vi "Problem1.14.vi"() -> ()   [LabVIEW 2019]
panel:
  in  "Begin Button":bool
  out "Current Element mod p":dbl
  out "Current Element":dbl
  out "Prime Array":dbl[](array[numeric])
  out "p":dbl
  out "Complete":bool
  out "Initial Array":dbl[](array[numeric])
  in  "Max Number":dbl
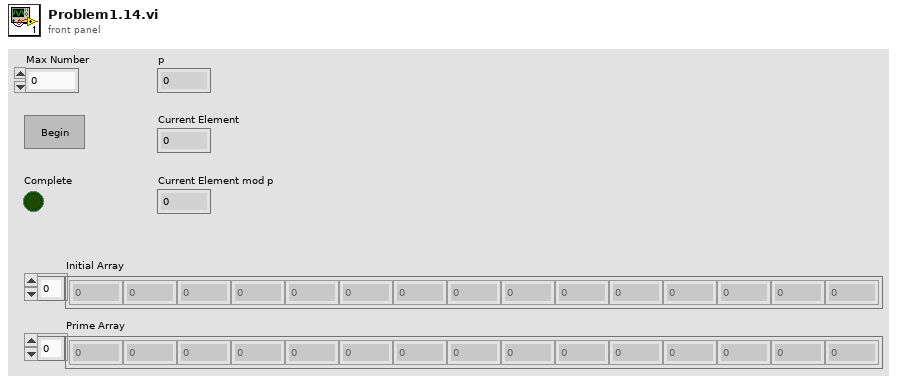
[diagram p1: front panel]
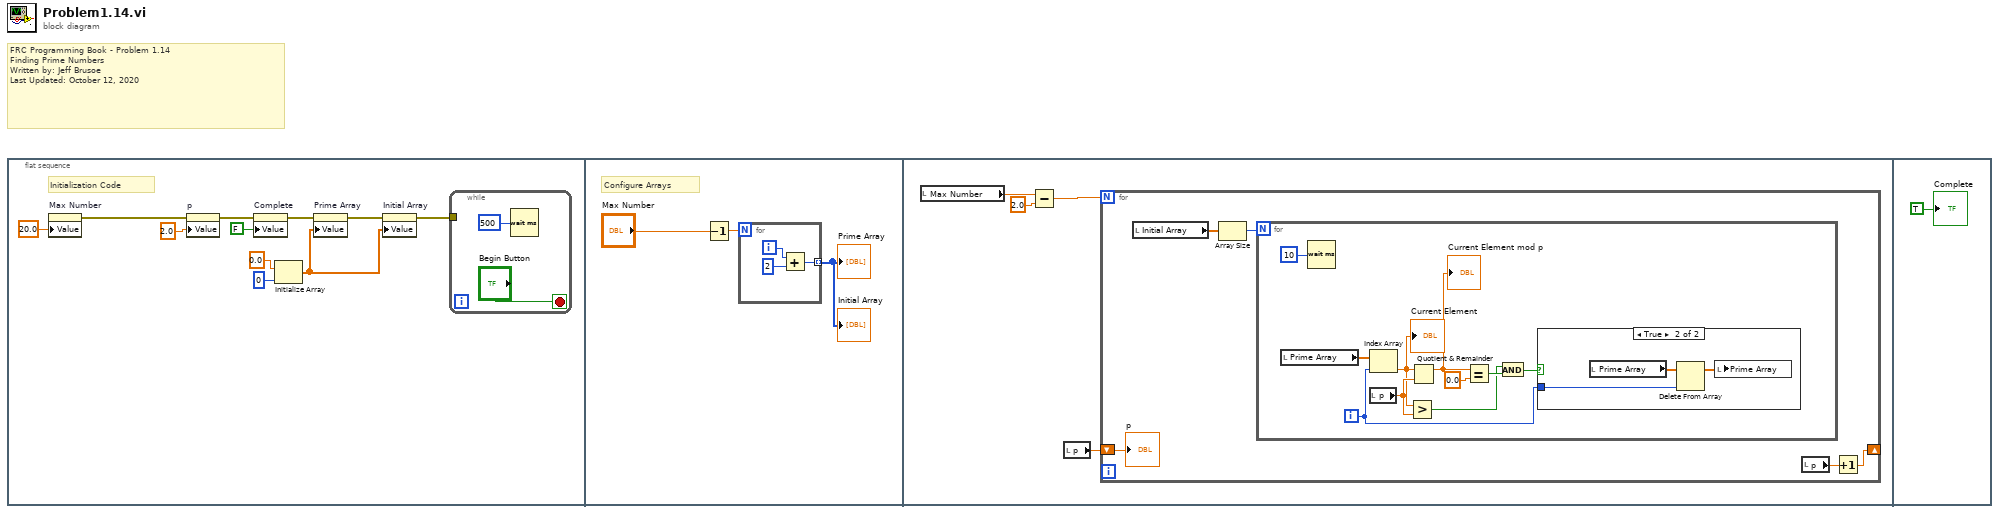
[diagram p0: block diagram]
diagram:
  # "FRC Programming Book - Problem 1.14\nFinding Prime Numbers\nWritten by: Jeff Brusoe\nLast Updated: October 12, 2020"
  n1 = flat-sequence {
    frame #0 {
      # "Initialization Code"
      n2 = property on="Max Number" class="DigNum (strict)"("Value"=20.0 ("Max Number")) -> (error out=w9:errorcluster)  [unwired: 2 in, 1 out]
      n3 = property on="p" class="DigNum (strict)"(error in=w9, "Value"=2.0 ("p")) -> (error out=w7:errorcluster)  [unwired: 1 in, 1 out]
      n4 = property on="Complete" class="Bool (strict)"(error in=w7, "Value"=FALSE ("Complete")) -> (error out=w4:errorcluster)  [unwired: 1 in, 1 out]
      n5 = Initialize Array(0.0 ("element"), 0 ("dimension size")) -> (w3:dbl[])
      n6 = property on="Prime Array" class="Arr (strict)"(error in=w4, "Value"=w3) -> (error out=w2:errorcluster)  [unwired: 1 in, 1 out]
      n7 = property on="Initial Array" class="Arr (strict)"(error in=w2, "Value"=w3) -> (error out=w1:errorcluster)  [unwired: 1 in, 1 out]
      n8 = while {
        tunnel: w1 -> [_]
        stop <- "Begin Button" stop-if-true
        n9 = Wait (ms)(milliseconds to wait=u32 500) -> ()  [unwired: 1 out]
      }
    }
    frame #1 {
      # "Configure Arrays"
      n10 = Decrement(x="Max Number") -> (x-1=w16:dbl)
      n11 = for {
        N: w16 -> [_]
        tunnel: [w17] -> w14 mode=indexing
        i -> [w19]
        n12 = Add(x=w19, y=2) -> (x+y=w17:i32)
      }
      "Initial Array" <- w14
      "Prime Array" <- w14
    }
    frame #2 {
      n13 = local read "Max Number"() -> (w21:dbl)
      n14 = Subtract(x=w21, y=2.0) -> (x-y=w22:dbl)
      n15 = local read "p"() -> (w23:dbl)
      n16 = for {
        N: w22 -> [_]
        shift-right: [w25] -> _
        shift-left: w23 -> [w26]
        n17 = local read "Initial Array"() -> (w27:dbl[])
        n18 = Array Size(array=w27) -> (size(s)=w28:i32)
        n19 = for {
          N: w28 -> [_]
          i -> [w29]
          n20 = local read "Prime Array"() -> (w38:dbl[])
          n21 = Wait (ms)(milliseconds to wait=u32 10) -> ()  [unwired: 1 out]
          n22 = Index Array(array=w38, index=w29) -> (element=w35:dbl)
          "Current Element" <- w35
          n23 = local read "p"() -> (w36:dbl)
          n24 = Greater?(x=w35, y=w36) -> (0:w31:bool)
          n25 = Quotient & Remainder(x=w35, y=w36) -> (x-y*floor(x/y)=w34:dbl)  [unwired: 1 out]
          "Current Element mod p" <- w34
          n26 = Equal?(x=w34, y=0.0) -> (x = y?=w32:bool)
          n27 = And(x=w31, y=w32) -> (x .and. y?=w30:bool)
          n28 = case shown="True" w30 {
            tunnel: w29 -> [_ w41]
            frame False {
            }
            frame True {
              n29 = local read "Prime Array"() -> (w40:dbl[])
              n30 = Delete From Array(array=w40, index=w41) -> (array with subset deleted=w39:dbl[])  [unwired: 1 in, 1 out]
              n31 = local write "Prime Array"(w39) -> ()
            }
          }
        }
        n32 = local read "p"() -> (w24:dbl)
        n33 = Increment(x=w24) -> (x+1=w25:dbl)
        "p" <- w26
      }
    }
    frame #3 {
      "Complete" <- TRUE ("Complete")
    }
  }
